vi "Pre-Run.vi"(8 "error in":errorcluster) -> (0 "error out":errorcluster)   [LabVIEW 2017, in "Logger.lvlib"]
uses:
  Logger.lvlib
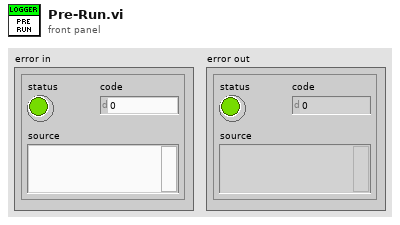
[diagram p1: front panel]
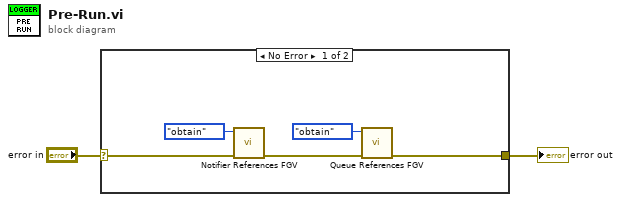
[diagram p0: block diagram]
diagram:
  n1 = case shown="No Error" "error in" {
    selector: "error in" -> [w7 w8]
    tunnel: [w5 w8] -> w1
    frame No Error {
      n2 = call "Notifier References FGV.vi"("error in"=w7, "function"=enum16{"obtain", "get", "release"}."obtain") -> ("error out"=w6:errorcluster)  [unwired: 8 in, 1 out]
      n3 = call "Queue References FGV.vi"("error in"=w6, "function"=enum16{"obtain", "get", "release"}."obtain") -> ("error out"=w5:errorcluster)  [unwired: 8 in, 1 out]
    }
    frame Error {
    }
  }
  "error out" <- w1
